vi "subElapsedTime_.vi"(0 "Reset":bool, 1 "Elapsed Time Target":dbl[](array[numeric]) format="%0.8f") -> (14 "Array":bool[](array[boolean]), 15 "Elapsed Time":dbl format="%0.2f")   [LabVIEW 2017]
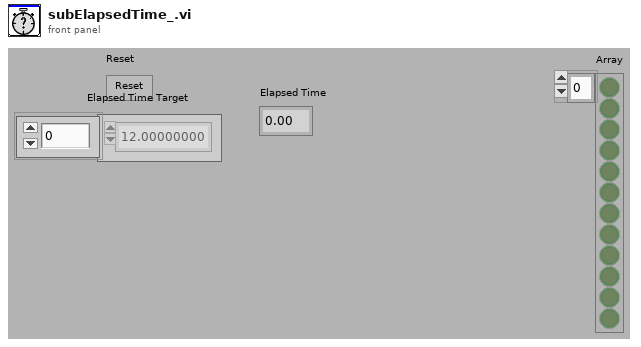
[diagram p1: front panel]
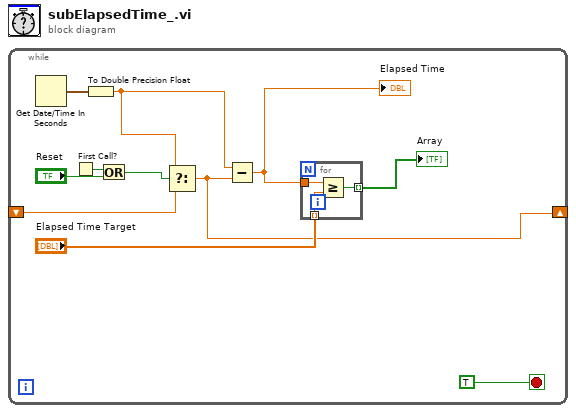
[diagram p0: block diagram]
diagram:
  n1 = while {
    shift-right: [w2] -> _
    shift-left: _ -> [w8]
    stop <- TRUE stop-if-true
    n2 = Get Date/Time In Seconds() -> (seconds since 1Jan1904=w5:timestamp)
    n3 = First Call?() -> (First Call?: T/F=w11:bool)
    n4 = To Double Precision Float(number=w5) -> (double precision float=w3:dbl)
    n5 = Or(x=w11, y="Reset") -> (x .or. y?=w4:bool)
    n6 = Select(t=w3, s=w4, f=w8) -> (s? t:f=w2:dbl)
    n7 = Subtract(x=w3, y=w2) -> (x-y=w6:dbl)
    "Elapsed Time" <- w6
    n8 = for {
      tunnel: "Elapsed Time Target" -> [w14] mode=indexing
      tunnel: [w13] -> w1 mode=indexing
      tunnel: w6 -> [w12]
      n9 = Greater Or Equal?(x=w12, y=w14) -> (x >= y?=w13:bool)
    }
    "Array" <- w1
  }
